vi "initialize.vi"(0 "HGF_DIMService":refnum<class "HGF_DIMService.lvclass">, 3 "initializationData":variant, 5 "error in (no error)":errorcluster, 7 "binaryString":string, 8 "I8 Array":i8[](array[numeric]), 9 "prependSize? (T)":bool, 11 "byteOrder (0:big-endian, network order)":T1(ring)) -> (14 "dup HGF_DIMService":refnum<class "HGF_DIMService.lvclass">, 17 "found?":bool, 19 "error out":errorcluster)   [LabVIEW 2012, in "HGF_DIM.lvlib" / "HGF_DIMService.lvclass"]
doc: "This is a dynamic dispatch VI to be implemented by child classes to initialize their attributes.\n\n<B>Recommendation:</B> Use Variant for initialization data."
uses:
  HGF_DIMService.lvclass
  HGF_BaseClasses/HGF_PVPublisher/HGF_PVPublisher.lvclass
  HGF_DIMService.lvclass/HGF_DIMService.ctl
  DimLVEvent/LVDimInterface/LVDimInterface.lvlib
  HGF_BaseClasses/HGF_Factory/HGF_Factory.lvclass
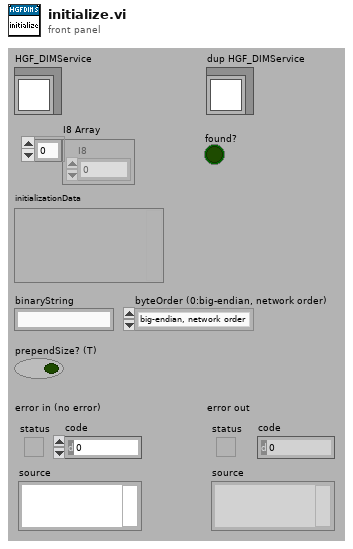
[diagram p1: front panel]
types:
  T1 = enum16{"big-endian, network order", "native, host order", "little-endian"}
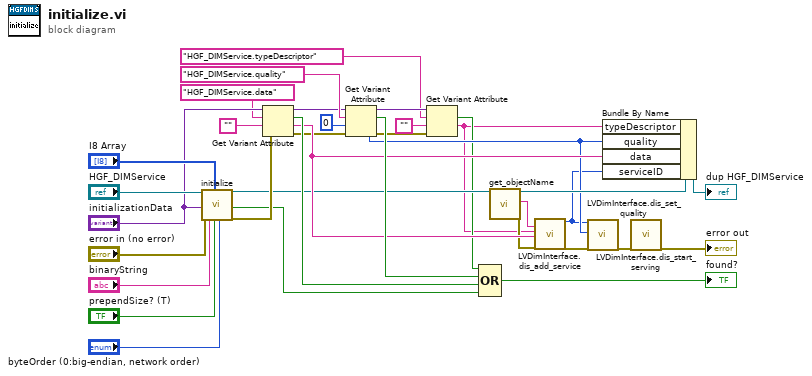
[diagram p0: block diagram]
diagram:
  n1 = call-parent "initialize.vi"("HGV_PVBase"="HGF_DIMService", "initializationData"="initializationData", "error in (no error)"="error in (no error)", "binaryString"="binaryString", "I8 Array"="I8 Array", "prependSize? (T)"="prependSize? (T)", "byteOrder (0:big-endian, network order)"="byteOrder (0:big-endian, network order)") -> ("HGV_PVBase"=w10:refnum<class "HGF_DIMService.lvclass">, "found?"=w21:bool, "error out"=w22:errorcluster)  [unwired: 10 out]
  n2 = Get Variant Attribute(Variant="initializationData", name="HGF_DIMService.data", default value (empty Variant)="", error in=w22) -> (duplicate Variant=w8:variant, found=w23:bool, value=w17:string, error out=w7:errorcluster)
  n3 = Get Variant Attribute(Variant=w8, name="HGF_DIMService.quality", default value (empty Variant)=0 ("quality"), error in=w7) -> (duplicate Variant=w6:variant, found=w24:bool, value=w14:i32, error out=w5:errorcluster)
  n4 = Get Variant Attribute(Variant=w6, name="HGF_DIMService.typeDescriptor", default value (empty Variant)="", error in=w5) -> (found=w2:bool, value=w1:string)  [unwired: 2 out]
  n5 = Compound Arithmetic op=OR(w2, w24, w23, w21) -> (→"found?":bool)
  n6 = call "get_objectName.vi"("HGF_Factory"=w10) -> ("dup HGF_Factory"=w19:refnum<class "HGF_DIMService.lvclass">, "objectName"=w18:string, "error out"=w16:errorcluster)  [unwired: 1 in, 15 out]
  n7 = call "LVDimInterface.dis_add_service.vi"("serviceName"=w18, "typeDescriptor"=w1, "data"=w17, "error in (no error)"=w16) -> ("my_serviceID"=w11:i32, "error out"=w15:errorcluster)  [unwired: 1 in, 13 out]
  n8 = call "LVDimInterface.dis_set_quality.vi"("my_serviceID"=w11, "quality"=w14, "error in (no error)"=w15) -> ("error out"=w13:errorcluster)  [unwired: 16 out]
  n9 = Bundle By Name(cluster=w19, "typeDescriptor"=w1, "quality"=w14, "data"=w17, "serviceID"=w11) -> (→"dup HGF_DIMService":refnum<class "HGF_DIMService.lvclass">)
  n10 = call "LVDimInterface.dis_start_serving.vi"("error in (no error)"=w13) -> ("error out"=→"error out":errorcluster)  [unwired: 1 in, 17 out]
